vi "Read configuration.vi"(8 "error in":errorcluster, 11 "Tagbus PID Module editor node in":refnum<class "PID Module editor node.lvclass">) -> (0 "error out":errorcluster, 2 "configuration":refnum<class "NISE_CEF_serializable configuration.lvclass">, 3 "Tagbus PID Module editor node out":refnum<class "PID Module editor node.lvclass">)   [LabVIEW 2014, in "PID Module editor node.lvclass"]
uses:
  PID Module editor node.lvclass
  <vilib>/NI/Configuration Framework/serializable configuration/NISE_CEF_serializable configuration.lvclass
  PID Module editor node.lvclass/PID Module editor node.ctl
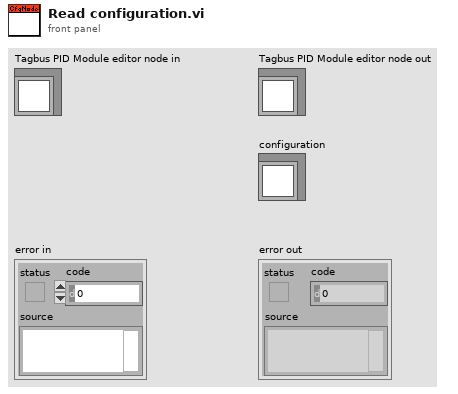
[diagram p1: front panel]
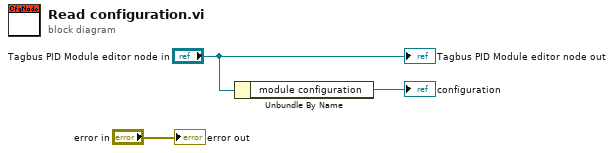
[diagram p0: block diagram]
diagram:
  n1 = Unbundle By Name("Tagbus PID Module editor node in") -> ("module configuration"=→"configuration":refnum<class "PID Module configuration.lvclass">)
  "error out" <- "error in"
  "Tagbus PID Module editor node out" <- "Tagbus PID Module editor node in"
